vi "Queue Driver.vi"(0 "Queue Ref In":refnum<queue>, 1 "Queue Name":string, 2 "State In":string, 3 "Data In":variant, 4 "EnqueueN States":string[](array[string]), 5 "error in (no error)":errorcluster, 9 "Queue Operation":T1) -> (14 "Queue Ref Out":refnum<queue>, 15 "State Out":string, 16 "Data Out":variant, 19 "error out":errorcluster)   [LabVIEW 2019, in "Queue Driver.lvlib"]
uses:
  Queue Driver.lvlib
  TypeDefs/Queue Operation.ctl
  TypeDefs/Queue Data.ctl
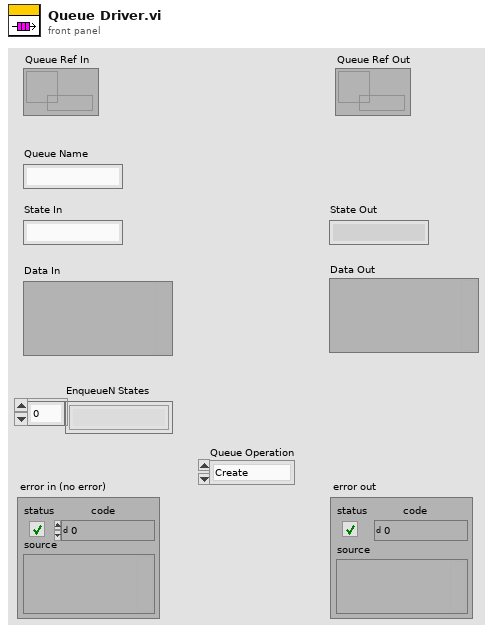
[diagram p1: front panel]
types:
  T1 = typedef "Queue Driver.lvlib/Queue Operation.ctl" = enum16{"Create", "Enqueue", "EnqueueN", "Dequeue", "Flush", "Destroy"}
  T2 = typedef "Queue Driver.lvlib/Queue Data.ctl" = cluster{"State":string, "Data":variant}
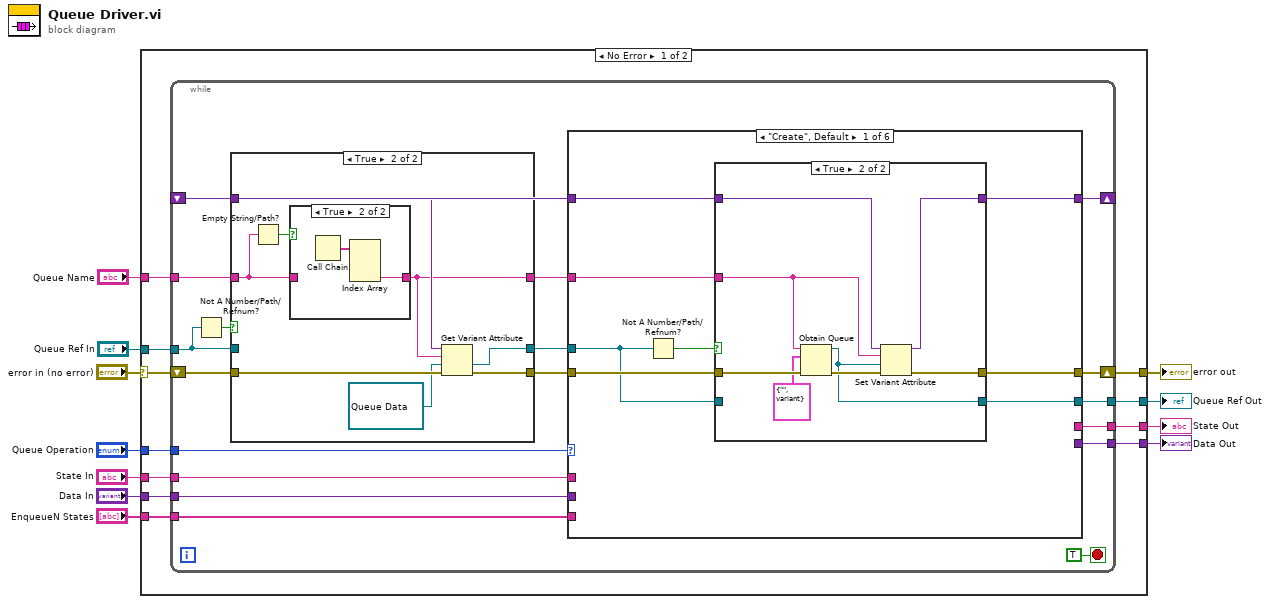
[diagram p0: block diagram]
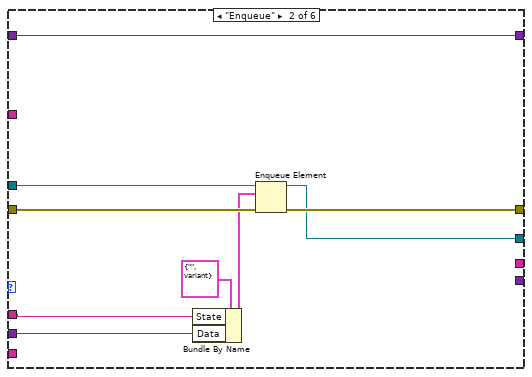
[diagram p5: hidden frame]
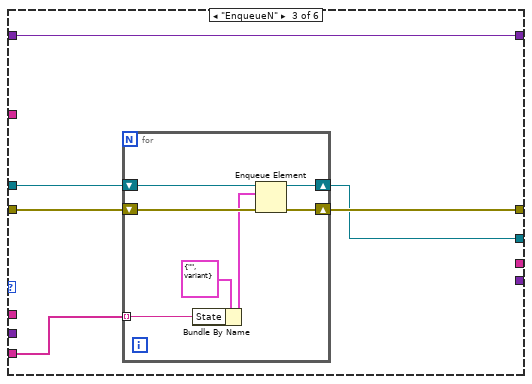
[diagram p6: hidden frame]
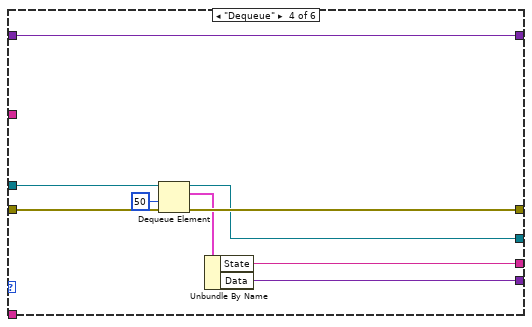
[diagram p7: hidden frame]
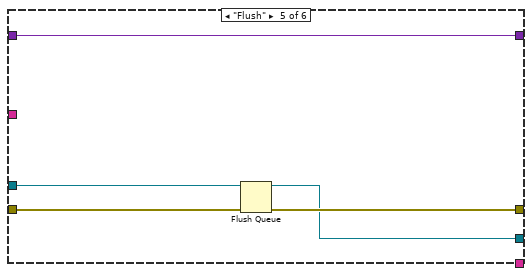
[diagram p8: hidden frame]
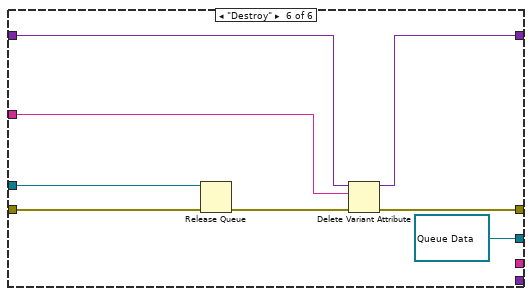
[diagram p9: hidden frame]
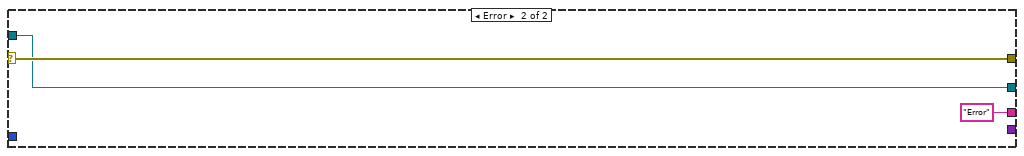
[diagram p10: hidden frame]
diagram:
  n1 = case shown="No Error" "error in (no error)" {
    selector: "error in (no error)" -> [w21 w119]
    tunnel: "Queue Operation" -> [w22 _]
    tunnel: "State In" -> [w20 _]
    tunnel: "Data In" -> [w19 _]
    tunnel: [w18 w119] -> w7
    tunnel: [w17 "Error" ("State")] -> w6
    tunnel: [w16 _] -> w5
    tunnel: "EnqueueN States" -> [w15 _]
    tunnel: "Queue Ref In" -> [w14 w117]
    tunnel: "Queue Name" -> [w13 _]
    tunnel: [w12 w117] -> w1
    frame No Error {
      n2 = while {
        tunnel: w22 -> [w40]
        shift-right: [w33] -> _
        shift-left: _ -> [w37]
        shift-right: [w34] -> w18
        shift-left: w21 -> [w38]
        tunnel: w20 -> [w31]
        tunnel: w19 -> [w30]
        tunnel: [w29] -> w17
        tunnel: [w28] -> w16
        tunnel: w15 -> [w27]
        tunnel: w14 -> [w25]
        tunnel: w13 -> [w24]
        tunnel: [w23] -> w12
        stop <- TRUE stop-if-true
        n3 = Not A Number/Path/Refnum?(number/path/refnum=w25) -> (NaN/Path/Refnum?=w26:bool)
        n4 = case shown="True" w26 {
          tunnel: [w41 w50] -> w39
          tunnel: w38 -> [w41 w49]
          tunnel: w37 -> [_ w48]
          tunnel: [w42 w46] -> w36
          tunnel: [_ w45] -> w35
          tunnel: w25 -> [w42 _]
          tunnel: w24 -> [_ w43]
          frame False {
          }
          frame True {
            n5 = Empty String/Path?(string/path=w43) -> (empty?=w44:bool)
            n6 = case shown="True" w44 {
              tunnel: [w51 w52] -> w45
              tunnel: w43 -> [w51 _]
              frame False {
              }
              frame True {
                n7 = Call Chain() -> (call chain=w53:string[])
                n8 = Index Array(array=w53) -> (element #3=w52:string)  [unwired: 3 in, 2 out]
              }
            }
            n9 = Get Variant Attribute(Variant=w48, name=w45, default value (empty Variant)=refnum<queue> refnum ("queue out"), error in=w49) -> (value=w46:refnum<queue>, error out=w50:errorcluster)  [unwired: 2 out]
          }
        }
        n10 = case shown="\"Create\", Default" w40 {
          tunnel: w39 -> [w61 w80 w86 w102 w106 w116]
          tunnel: w37 -> [w57 w81 w87 w103 w108 w111]
          tunnel: w36 -> [w54 w79 w85 w101 w105 w115]
          tunnel: w35 -> [w59 _ _ _ _ w110]
          tunnel: [w58 w74 w84 w100 w107 w113] -> w34
          tunnel: [w56 w81 w87 w103 w108 w112] -> w33
          tunnel: w31 -> [_ w77 _ _ _ _]
          tunnel: w30 -> [_ w76 _ _ _ _]
          tunnel: [_ _ _ w98 _ _] -> w29
          tunnel: [_ _ _ w97 _ _] -> w28
          tunnel: w27 -> [_ _ w83 _ _ _]
          tunnel: [w55 w73 w82 w95 w104 refnum<queue> refnum ("queue out")] -> w23
          frame "Create", Default {
            n11 = Not A Number/Path/Refnum?(number/path/refnum=w54) -> (NaN/Path/Refnum?=w60:bool)
            n12 = case shown="True" w60 {
              tunnel: w61 -> [w64 w72]
              tunnel: w59 -> [_ w67]
              tunnel: [w64 w69] -> w58
              tunnel: w57 -> [w63 w68]
              tunnel: [w63 w66] -> w56
              tunnel: [w62 w65] -> w55
              tunnel: w54 -> [w62 _]
              frame False {
              }
              frame True {
                n13 = Obtain Queue(name (unnamed)=w67, element data type=T2 {"State"="", "Data"=variant} ("Queue Data"), error in (no error)=w72) -> (queue out=w65:refnum<queue>, error out=w70:errorcluster)  [unwired: 2 in, 1 out]
                n14 = Set Variant Attribute(Variant=w68, name=w67, value=w65, error in=w70) -> (Variant out=w66:variant, error out=w69:errorcluster)  [unwired: 1 out]
              }
            }
          }
          frame "Enqueue" {
            n15 = Bundle By Name(cluster=T2 {"State"="", "Data"=variant} ("Queue Data"), "State"=w77, "Data"=w76) -> (w75:T2)
            n16 = Enqueue Element(queue=w79, element=w75, error in (no error)=w80) -> (queue out=w73:refnum<queue>, error out=w74:errorcluster)  [unwired: 1 in, 1 out]
          }
          frame "EnqueueN" {
            n17 = for {
              shift-right: [w90] -> w84
              shift-left: w86 -> [w94]
              tunnel: w83 -> [w89] mode=indexing
              shift-right: [w88] -> w82
              shift-left: w85 -> [w93]
              n18 = Bundle By Name(cluster=T2 {"State"="", "Data"=variant} ("Queue Data"), "State"=w89) -> (w91:T2)
              n19 = Enqueue Element(queue=w93, element=w91, error in (no error)=w94) -> (queue out=w88:refnum<queue>, error out=w90:errorcluster)  [unwired: 1 in, 1 out]
            }
          }
          frame "Dequeue" {
            n20 = Dequeue Element(queue=w101, timeout in ms (-1)=50, error in (no error)=w102) -> (queue out=w95:refnum<queue>, element=w99:T2, error out=w100:errorcluster)  [unwired: 1 out]
            n21 = Unbundle By Name(w99) -> ("State"=w98:string, "Data"=w97:variant)
          }
          frame "Flush" {
            n22 = Flush Queue(queue=w105, error in (no error)=w106) -> (queue out=w104:refnum<queue>, error out=w107:errorcluster)  [unwired: 1 out]
          }
          frame "Destroy" {
            n23 = Release Queue(queue=w115, error in (no error)=w116) -> (error out=w114:errorcluster)  [unwired: 1 in, 2 out]
            n24 = Delete Variant Attribute(4:w114, 6:w110, 7:w111) -> (0:w113:errorcluster, 3:w112:variant)  [unwired: 1 out]
          }
        }
      }
    }
    frame Error {
    }
  }
  "error out" <- w7
  "State Out" <- w6
  "Data Out" <- w5
  "Queue Ref Out" <- w1
